vi "Start Boiler.vi"(7 "Log File Refnum in":refnum<file>, 8 "error in":errorcluster, 9 "UI Data in":T2, 10 "Handshake Notifier in":refnum<notifier>, 11 "Message Queues in":T1) -> (0 "error out":errorcluster, 1 "UI Data out":T2, 2 "Handshake Notifier out":refnum<notifier>, 3 "Message Queues out":T1, 5 "Log File Refnum out":refnum<file>)   [LabVIEW 2017, in "Controller.lvlib"]
doc: "Start the flow of hot air from the boiler."
uses:
  Controller.lvlib
  controls/MHL UI Data.ctl
  controls/MHL Status.ctl
  support/Message Queue/All Message Queues.ctl
  support/Message Queue/Message Cluster.ctl
  support/Boiler System Globals.vi
  support/Message Queue/Message Queue.lvlib
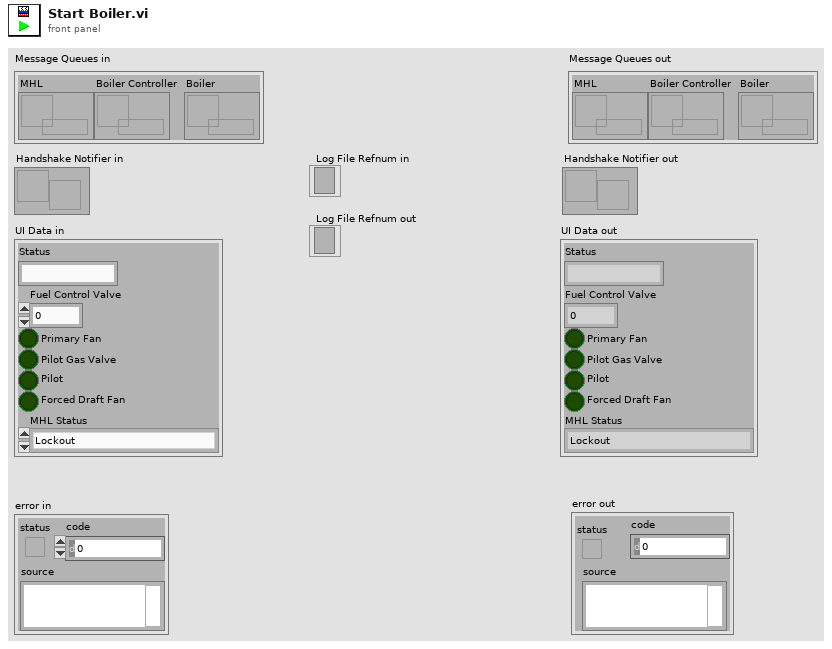
[diagram p1: front panel]
types:
  T1 = typedef "Message Queue.lvlib/All Message Queues.ctl" = cluster{"MHL":refnum<queue>, "Boiler Controller":refnum<queue>, "Boiler":refnum<queue>}
  T2 = typedef "MHL UI Data.ctl" = cluster{"Status":string, "Fuel Control Valve":u32, "Primary Fan":bool, "Pilot Gas Valve":bool, "Pilot":bool, "Forced Draft Fan":bool, "MHL Status":T3}
  T3 = typedef "MHL Status.ctl" = enum16{"Lockout", "Ready", "Pre-Purge", "Pre-Purge Complete", "Pilot On", "Boiler Running", "Shutdown", "Purge"}
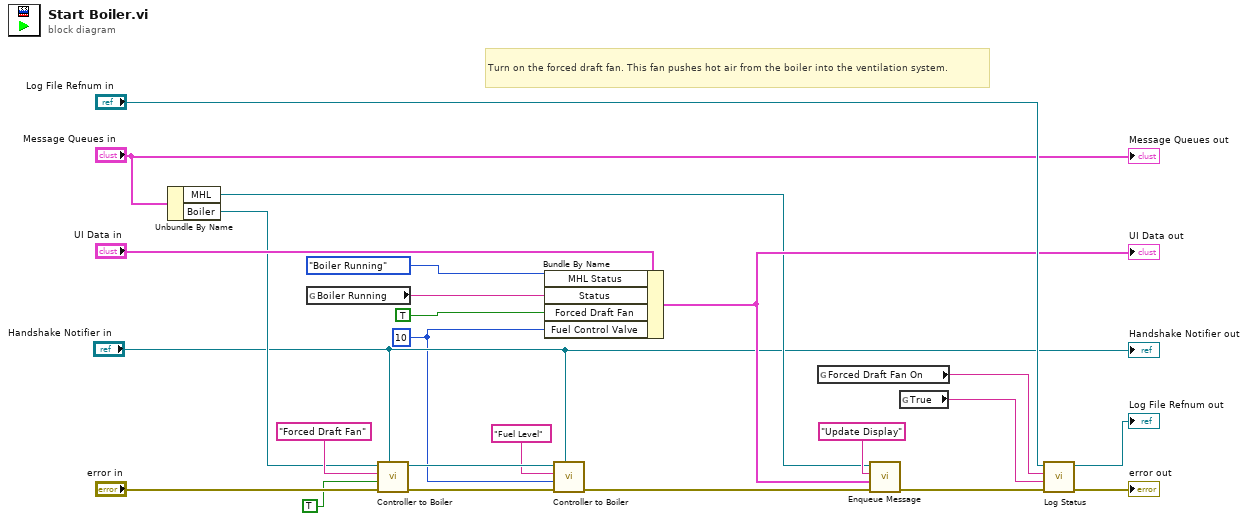
[diagram p0: block diagram]
diagram:
  w3 = u32 10 ("Fuel Control Valve")
  # "Turn on the forced draft fan. This fan pushes hot air from the boiler into the ventilation system."
  n1 = Unbundle By Name("Message Queues in") -> ("MHL"=w13:refnum<queue>, "Boiler"=w12:refnum<queue>)
  n2 = global read "Boiler System Globals.vi" "Boiler Running"() -> (w9:string)
  n3 = call "Controller to Boiler.vi"("Notifier"="Handshake Notifier in", "error in"="error in", "Message Data"=TRUE, "Message"="Forced Draft Fan", "Boiler Queue in"=w12) -> ("error out"=w8:errorcluster, "Queue out"=w5:refnum<queue>)  [unwired: 4 in, 1 out]
  n4 = Bundle By Name(cluster="UI Data in", "MHL Status"=MHL_Status."Boiler Running", "Status"=w9, "Forced Draft Fan"=TRUE, "Fuel Control Valve"=w3) -> (w18:T2)
  "UI Data out" <- w18
  n5 = call "Controller to Boiler.vi"("Notifier"="Handshake Notifier in", "error in"=w8, "Message Data"=w3, "Message"="Fuel Level", "Boiler Queue in"=w5) -> ("error out"=w7:errorcluster)  [unwired: 4 in, 2 out]
  n6 = global read "Boiler System Globals.vi" "Forced Draft Fan On"() -> (w10:string)
  n7 = call "Enqueue Message.vi"("error in (no error)"=w7, "Message Data"=w18, "Message"="Update Display", "Message Queue"=w13) -> ("error out"=w19:errorcluster)  [unwired: 6 in, 1 out]
  n8 = global read "Boiler System Globals.vi" "True"() -> (w11:string)
  n9 = call "Log Status.vi"("error in"=w19, "Event Data String (-)"=w11, "Event String"=w10, "Log File Refnum In"="Log File Refnum in") -> ("error out"=→"error out":errorcluster, "Log File Refnum Out"=→"Log File Refnum out":refnum<file>)  [unwired: 6 in]
  "Message Queues out" <- "Message Queues in"
  "Handshake Notifier out" <- "Handshake Notifier in"
